vi "update the test result table_bakcup.vi"(6 "Bool引用句柄":refnum<vi>, 7 "Test Result":string[](array[string]), 8 "数组":string[][](array[string]), 9 "Test Start Time":string, 10 "Test Table":refnum<vi>, 11 "LED":T1) -> ()   [LabVIEW 2016]
uses:
  <vilib>/Utility/miscctls.llb/LVRowAndColumnTypeDef.ctl
  Global Variables/Pacemaker ASIC Test_Save_SN Globals.vi
  Global Variables/Pacemaker ASIC Test_Config Globals.vi
  <vilib>/Utility/file.llb/Write Delimited Spreadsheet (string).vi
panel:
  in  "Test Unit Information":string[][](array[string])=[["Module", "SRN"], ["Software", "V01"]]
  in  "清除原有数据":bool
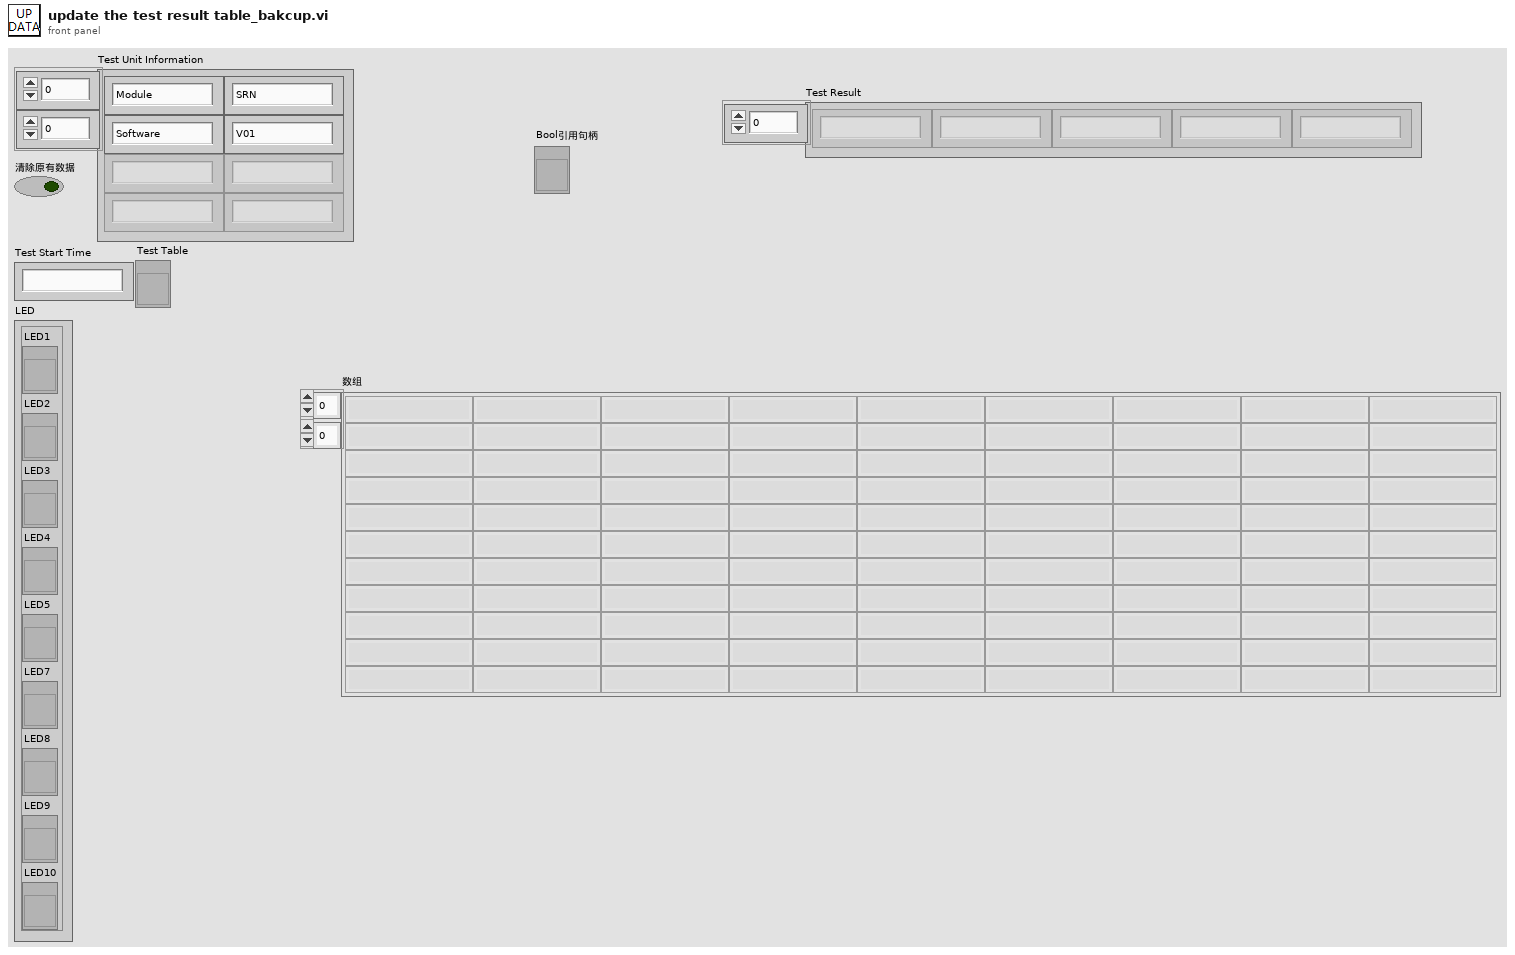
[diagram p1: front panel]
types:
  T1 = cluster{"LED1":refnum<vi>, "LED2":refnum<vi>, "LED3":refnum<vi>, "LED4":refnum<vi>, "LED5":refnum<vi>, "LED7":refnum<vi>, "LED8":refnum<vi>, "LED9":refnum<vi>, "LED10":refnum<vi>}
  T2 = typedef "LVRowAndColumnTypeDef.ctl" = cluster{"Row":i32, "Column":i32}
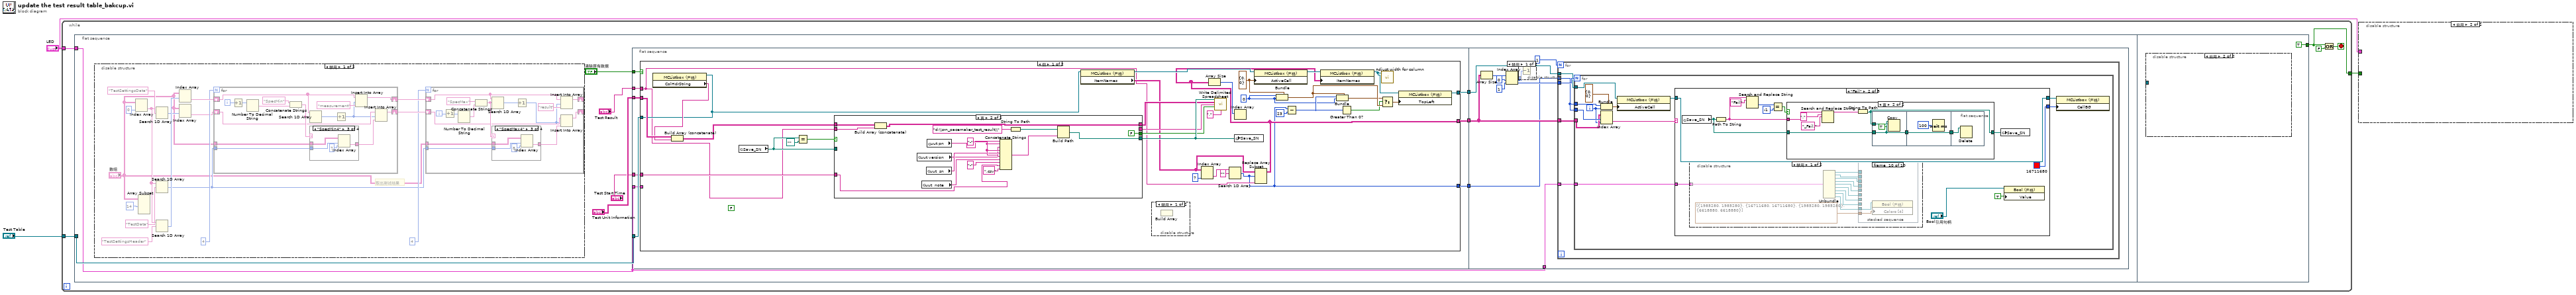
[diagram p0: block diagram]
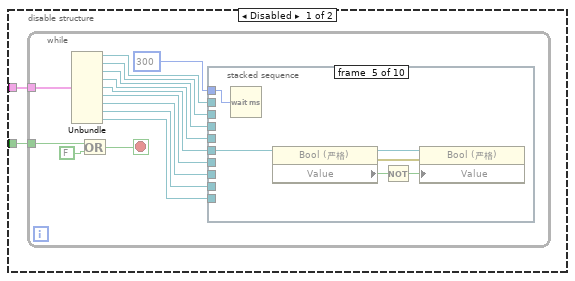
[diagram p2: hidden frame]
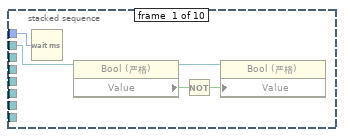
[diagram p3: hidden frame]
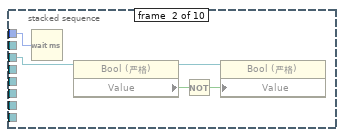
[diagram p4: hidden frame]
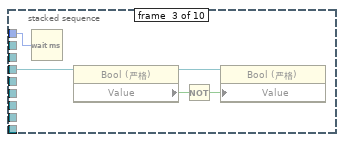
[diagram p5: hidden frame]
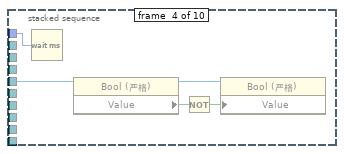
[diagram p6: hidden frame]
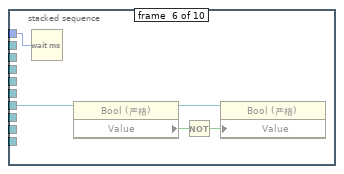
[diagram p7: hidden frame]
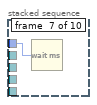
[diagram p8: hidden frame]
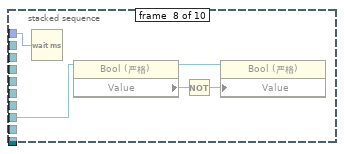
[diagram p9: hidden frame]
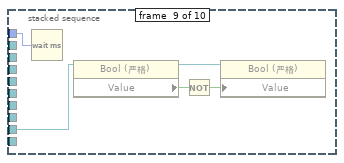
[diagram p10: hidden frame]
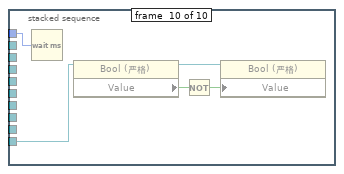
[diagram p11: hidden frame]
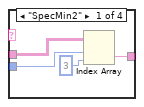
[diagram p12: hidden frame]
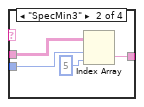
[diagram p13: hidden frame]
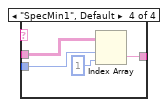
[diagram p14: hidden frame]
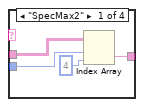
[diagram p15: hidden frame]
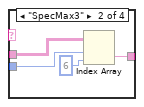
[diagram p16: hidden frame]
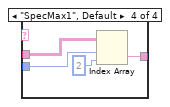
[diagram p17: hidden frame]
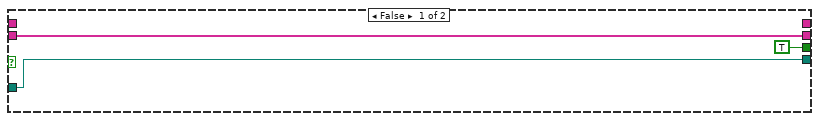
[diagram p20: hidden frame]
diagram:
  n1 = while {
    tunnel: "Test Table" -> [w8]
    tunnel: [w5] -> w3
    tunnel: "LED" -> [w4]
    stop <- w6 stop-if-true
    n2 = flat-sequence {
      tunnel: w8 -> [w14]
      tunnel: w4 -> [w13]
      tunnel: [TRUE] -> w5
      frame #0 {
        n3 = disable-structure shown="禁用" {
          frame Disabled {
            # "取出测试结果"
            n4 = Index Array(array="数组", index (col)=0 ("禁用的索引 (列)")) -> (element=w22:string[])  [unwired: 1 in]
            n5 = Array Subset(array="数组", length (row)=14 ("长度")) -> ()  [unwired: 3 in, 1 out]
            n6 = Search 1D Array(1D array=w22, element="TestSettingsData" ("元素")) -> (index of element=w23:i32)  [unwired: 1 in]
            n7 = Search 1D Array(1D array=w22, element="TestData" ("元素")) -> (index of element=w20:i32)  [unwired: 1 in]
            n8 = Search 1D Array(1D array=w22, element="TestSettingsHeader" ("元素")) -> (index of element=w25:i32)  [unwired: 1 in]
            n9 = Index Array(array="数组", index (row)=w25) -> (element=w33:string[])  [unwired: 1 in]
            n10 = Index Array(array="数组", index (row)=w23) -> (element=w31:string[])  [unwired: 1 in]
            n11 = for {
              N: 4 -> [_]
              shift-right: [w42] -> w30
              shift-left: w33 -> [w43]
              shift-right: [w39] -> w29
              shift-left: w31 -> [w40]
              tunnel: "数组" -> [w35]
              tunnel: w20 -> [w34]
              i -> [w47]
              n12 = Increment(x=w47) -> (x+1=w46:i32)
              n13 = Number To Decimal String(number=w46) -> (decimal integer string=w45:string)  [unwired: 1 in]
              n14 = Concatenate Strings("SpecMin" ("元素"), w45) -> (w44:string)
              n15 = Search 1D Array(1D array=w43, element=w44) -> (index of element=w41:i32)  [unwired: 1 in]
              n16 = case shown="\"SpecMin4\"" w44 {
                tunnel: w35 -> [w51 w55 w57 w64]
                tunnel: [w50 w53 w59 w62] -> w37
                tunnel: w34 -> [w49 w54 w58 w61]
                frame "SpecMin2" {
                  n17 = Index Array(array=w51, index (row)=w49, index (col)=3) -> (element=w50:string)
                }
                frame "SpecMin3" {
                  n18 = Index Array(array=w55, index (row)=w54, index (col)=5) -> (element=w53:string)
                }
                frame "SpecMin4" {
                  n19 = Index Array(array=w57, index (row)=w58, index (col)=7) -> (element=w59:string)
                }
                frame "SpecMin1", Default {
                  n20 = Index Array(array=w64, index (row)=w61, index (col)=1) -> (element=w62:string)
                }
              }
              n21 = Increment(x=w41) -> (x+1=w36:i32)
              n22 = Insert Into Array(array=w43, index=w36, new element="measurement" ("新元素/子数组")) -> (w42:string[])
              n23 = Insert Into Array(array=w40, index=w36, new element=w37) -> (w39:string[])
            }
            n24 = for {
              N: 4 -> [_]
              shift-right: [w73] -> _
              shift-left: w30 -> [w74]
              shift-right: [w70] -> _
              shift-left: w29 -> [w71]
              tunnel: "数组" -> [w66]
              tunnel: w20 -> [w65]
              i -> [w78]
              n25 = Increment(x=w78) -> (x+1=w77:i32)
              n26 = Number To Decimal String(number=w77) -> (decimal integer string=w76:string)  [unwired: 1 in]
              n27 = Concatenate Strings("SpecMax" ("元素"), w76) -> (w75:string)
              n28 = Search 1D Array(1D array=w74, element=w75) -> (index of element=w72:i32)  [unwired: 1 in]
              n29 = case shown="\"SpecMax4\"" w75 {
                tunnel: w66 -> [w82 w86 w89 w95]
                tunnel: [w81 w84 w90 w93] -> w68
                tunnel: w65 -> [w80 w85 w88 w92]
                frame "SpecMax2" {
                  n30 = Index Array(array=w82, index (row)=w80, index (col)=4) -> (element=w81:string)
                }
                frame "SpecMax3" {
                  n31 = Index Array(array=w86, index (row)=w85, index (col)=6) -> (element=w84:string)
                }
                frame "SpecMax4" {
                  n32 = Index Array(array=w89, index (row)=w88, index (col)=8) -> (element=w90:string)
                }
                frame "SpecMax1", Default {
                  n33 = Index Array(array=w95, index (row)=w92, index (col)=2) -> (element=w93:string)
                }
              }
              n34 = Increment(x=w72) -> (x+1=w67:i32)
              n35 = Insert Into Array(array=w74, index=w67, new element="result" ("新元素/子数组")) -> (w73:string[])
              n36 = Insert Into Array(array=w71, index=w67, new element=w68) -> (w70:string[])
            }
          }
          frame Enabled {
          }
        }
        n37 = flat-sequence {
          tunnel: "Test Result" -> [w104]
          tunnel: "清除原有数据" -> [w103]
          tunnel: w14 -> [w102]
          tunnel: [w101] -> w17
          tunnel: [w100] -> w16
          tunnel: w13 -> [w99]
          tunnel: "Test Unit Information" -> [w98]
          tunnel: "Test Start Time" -> [w97]
          tunnel: [w96] -> w9
          tunnel: w17 -> [w243]
          tunnel: w16 -> [w242]
          tunnel: w13 -> [w241]
          tunnel: w9 -> [w238]
          frame #0 {
            n38 = case shown="假" w103 {
              tunnel: w104 -> [w107 _]
              tunnel: w102 -> [w112 w179]
              tunnel: [w106 _] -> w101
              tunnel: [w121 w177] -> w100
              tunnel: w99 -> [_ w176]
              tunnel: w98 -> [w134 _]
              tunnel: w97 -> [w113 _]
              tunnel: [w105 _] -> w96
              frame False {
                (unwired) FALSE
                w116 = 0
                w125 = T2 {"Row"=0, "Column"=0} ("活动单元格:活动单元格")
                n39 = property class="MCListbox (严格)"(reference=w112) -> ("ColHdrString"=w114:string[])  [unwired: 1 in, 2 out]
                n40 = Build Array (concatenate)(w134, w114) -> (w135:string[][])
                n41 = global read "Pacemaker ASIC Test_Save_SN Globals.vi" "Save_SN"() -> (w131:path)
                n42 = Equal?(x=w131, y=path "") -> (x = y?=w132:bool)
                n43 = case shown="真" w132 {
                  tunnel: w135 -> [_ w144]
                  tunnel: w131 -> [w140 _]
                  tunnel: [w140 w146] -> w130
                  tunnel: [_ w142] -> w129
                  tunnel: [TRUE FALSE] -> w128
                  tunnel: w107 -> [w138 w143]
                  tunnel: [w138 _] -> w127
                  tunnel: w113 -> [_ w141]
                  frame False {
                  }
                  frame True {
                    w155 = "-"
                    n44 = Build Array (concatenate)(w144, w143) -> (w142:string[][])
                    n45 = global read "Pacemaker ASIC Test_Config Globals.vi" "uut version"() -> (w153:string)
                    n46 = global read "Pacemaker ASIC Test_Config Globals.vi" "uut  note"() -> (w156:string)
                    n47 = global read "Pacemaker ASIC Test_Config Globals.vi" "uut  sn"() -> (w154:string)
                    n48 = global read "Pacemaker ASIC Test_Config Globals.vi" "uut pn"() -> (w152:string)
                    n49 = Concatenate Strings(w152, w155, w153, w155, w154, w155, w156, "-", w141, ".csv" ("字符串")) -> (w148:string)
                    n50 = String To Path(string="d:\\srn_pacemaker_test_result\\" ("字符串")) -> (path=w149:path)
                    n51 = Build Path(base path=w149, name or relative path=w148) -> (appended path=w146:path)
                  }
                }
                n52 = property class="MCListbox (严格)"(reference=w112) -> (reference out=w136:refnum<vi>, "ItemNames"=w108:string[][])  [unwired: 1 in, 1 out]
                n53 = disable-structure shown="禁用" {
                  frame Disabled {
                    n54 = Build Array() -> ()  [unwired: 2 in, 1 out]
                  }
                  frame Enabled {
                  }
                }
                n55 = Index Array(array=w108, index (col)=7 ("禁用的索引 (列)")) -> (element=w110:string[])  [unwired: 1 in]
                n56 = call-poly <vilib>:"Write Delimited Spreadsheet.vi"("file path (dialog if empty)"=w130, "2D data"=w129, "1D data"=w127, "append to file? (new file:F)"=w128, "delimiter (\\t)"="," ("delimiter (\\t)")) -> ()  [unwired: 9 in, 2 out]
                n57 = Search 1D Array(1D array=w110, element="" ("元素")) -> (index of element=w105:i32)  [unwired: 1 in]
                n58 = global write "Pacemaker ASIC Test_Save_SN Globals.vi" "Save_SN"(w130) -> ()
                n59 = property class="MCListbox (严格)"(reference=w136, "ActiveCell"=w125) -> (reference out=w137:refnum<vi>)  [unwired: 1 in, 1 out]
                n60 = Replace Array Subset(array=w108, new element=w107, index (row)=w105) -> (w106:string[][])  [unwired: 1 in]
                n61 = Array Size(array=w106) -> (size(s)=w126:i32[])
                n62 = Index Array(array=w126) -> ()  [unwired: 1 in, 1 out]
                n63 = Bundle(cluster=w125, "Row"=w116, "Column"=w116) -> (w124:T2)
                n64 = Subtract(x=w105, y=23) -> (x-y=w117:i32)
                n65 = property class="MCListbox (严格)"(reference=w137, "ItemNames"=w106) -> (reference out=w120:refnum<vi>)  [unwired: 1 in, 1 out]
                n66 = Bundle(cluster=w124, "Row"=w117, "Column"=w116) -> (w123:T2)
                n67 = Greater Than 0?(x=w117) -> (x > 0?=w118:bool)
                n68 = call "Adjust width for column.vi"("MCListbox引用句柄"=w120) -> ()  [unwired: 11 in]
                n69 = Select(t=w123, s=w118, f=w124) -> (s? t:f=w122:T2)
                n70 = property class="MCListbox (严格)"(reference=w120, "TopLeft"=w122) -> (reference out=w121:refnum<vi>)  [unwired: 1 in, 1 out]
              }
              frame True {
                # "初始化MCListbox到空"
                n71 = property class="MCListbox (严格)"(reference=w179, "ActiveCell"=T2 {"Row"=0, "Column"=0} ("活动单元格:活动单元格")) -> (reference out=w164:refnum<vi>)  [unwired: 1 in, 1 out]
                n72 = property class="MCListbox (严格)"(reference=w164) -> (reference out=w163:refnum<vi>, "ItemNames"=w162:string[][])  [unwired: 1 in, 1 out]
                n73 = Array Size(array=w162) -> (size(s)=w161:i32[])
                n74 = property class="MCListbox (严格)"(reference=w163, "ItemNames"=string[][] [] ("项名")) -> (reference out=w178:refnum<vi>)  [unwired: 1 in, 1 out]
                n75 = Index Array(array=w161, index #1=0 ("索引"), index #2=1 ("索引")) -> (element #1=w159:i32, element #2=w157:i32)
                n76 = for {
                  N: w159 -> [_]
                  tunnel: w178 -> [w224]
                  tunnel: [w223] -> w177
                  tunnel: w157 -> [w222]
                  i -> [w225]
                  n77 = for {
                    N: w222 -> [_]
                    tunnel: w225 -> [w232]
                    tunnel: w224 -> [w229]
                    tunnel: [w228] -> w223
                    i -> [w231]
                    n78 = Bundle(cluster=cluster{i32, i32} {0, 0} ("簇"), w232, w231) -> (w233:cluster{i32, i32})
                    n79 = property class="MCListbox (严格)"(reference=w229, "ActiveCell"=w233) -> (reference out=w226:refnum<vi>)  [unwired: 1 in, 1 out]
                    n80 = disable-structure shown="启用" {
                      disable-tunnel: w226 -> [w236 _]
                      disable-tunnel: [w235 _] -> _
                      disable-tunnel: [w234 _] -> _
                      frame Disabled {
                        n81 = property class="MCListbox (严格)"(reference=w236) -> (reference out=w235:refnum<vi>, "CellBG"=w237:u32)  [unwired: 1 in, 1 out]
                        n82 = Not Equal?(x=w237) -> (x != y?=w234:bool)  [unwired: 1 in]
                      }
                      frame Enabled {
                      }
                    }
                    n83 = property class="MCListbox (严格)"(reference=w226, "CellBG"=u32 16448250) -> (reference out=w228:refnum<vi>)  [unwired: 1 in, 1 out]
                  }
                }
                n84 = Unbundle(w176) -> ("LED1"=w175:refnum<vi>, "LED2"=w174:refnum<vi>, "LED3"=w173:refnum<vi>, "LED4"=w172:refnum<vi>, "LED5"=w171:refnum<vi>, "LED7"=w170:refnum<vi>, "LED8"=w167:refnum<vi>, "LED9"=w168:refnum<vi>, "LED10"=w169:refnum<vi>)
                n85 = stacked-sequence {
                  tunnel: w175 -> [w185 _ _ _ _ _ _ _ _ _]
                  tunnel: w174 -> [_ w189 _ _ _ _ _ _ _ _]
                  tunnel: w173 -> [_ _ w193 _ _ _ _ _ _ _]
                  tunnel: w172 -> [_ _ _ w197 _ _ _ _ _ _]
                  tunnel: w171 -> [_ _ _ _ w201 _ _ _ _ _]
                  tunnel: w170 -> [_ _ _ _ _ w205 _ _ _ _]
                  tunnel: w169 -> [_ _ _ _ _ _ _ _ _ w221]
                  tunnel: w168 -> [_ _ _ _ _ _ _ _ w216 _]
                  tunnel: w167 -> [_ _ _ _ _ _ w209 w213 _ _]
                  tunnel: cluster{u32, u32}[] [{1985280, 1985280}, {65358, 65358}, {1985280, 1985280}, {6618880, 6618880}] ("颜色[4]") -> [w184 w188 w192 w196 w200 w204 w208 w212 w217 w220]
                  tunnel: TRUE -> [w183 w187 w191 w194 w198 w202 w206 w210 w214 w218]
                  frame #0 {
                    n86 = property class="Bool (严格)"(reference=w185, "Colors [4]"=w184) -> (reference out=w182:refnum<vi>)  [unwired: 1 in, 1 out]
                    n87 = property class="Bool (严格)"(reference=w182, "Value"=w183) -> ()  [unwired: 1 in, 2 out]
                  }
                  frame #1 {
                    n88 = property class="Bool (严格)"(reference=w189, "Colors [4]"=w188) -> (reference out=w186:refnum<vi>)  [unwired: 1 in, 1 out]
                    n89 = property class="Bool (严格)"(reference=w186, "Value"=w187) -> ()  [unwired: 1 in, 2 out]
                  }
                  frame #2 {
                    n90 = property class="Bool (严格)"(reference=w193, "Colors [4]"=w192) -> (reference out=w190:refnum<vi>)  [unwired: 1 in, 1 out]
                    n91 = property class="Bool (严格)"(reference=w190, "Value"=w191) -> ()  [unwired: 1 in, 2 out]
                  }
                  frame #3 {
                    n92 = property class="Bool (严格)"(reference=w197, "Colors [4]"=w196) -> (reference out=w195:refnum<vi>)  [unwired: 1 in, 1 out]
                    n93 = property class="Bool (严格)"(reference=w195, "Value"=w194) -> ()  [unwired: 1 in, 2 out]
                  }
                  frame #4 {
                    n94 = property class="Bool (严格)"(reference=w201, "Colors [4]"=w200) -> (reference out=w199:refnum<vi>)  [unwired: 1 in, 1 out]
                    n95 = property class="Bool (严格)"(reference=w199, "Value"=w198) -> ()  [unwired: 1 in, 2 out]
                  }
                  frame #5 {
                    n96 = property class="Bool (严格)"(reference=w205, "Colors [4]"=w204) -> (reference out=w203:refnum<vi>)  [unwired: 1 in, 1 out]
                    n97 = property class="Bool (严格)"(reference=w203, "Value"=w202) -> ()  [unwired: 1 in, 2 out]
                  }
                  frame #6 {
                    n98 = property class="Bool (严格)"(reference=w209, "Colors [4]"=w208) -> (reference out=w207:refnum<vi>)  [unwired: 1 in, 1 out]
                    n99 = property class="Bool (严格)"(reference=w207, "Value"=w206) -> ()  [unwired: 1 in, 2 out]
                  }
                  frame #7 {
                    n100 = property class="Bool (严格)"(reference=w213, "Colors [4]"=w212) -> (reference out=w211:refnum<vi>)  [unwired: 1 in, 1 out]
                    n101 = property class="Bool (严格)"(reference=w211, "Value"=w210) -> ()  [unwired: 1 in, 2 out]
                  }
                  frame #8 {
                    n102 = property class="Bool (严格)"(reference=w216, "Colors [4]"=w217) -> (reference out=w215:refnum<vi>)  [unwired: 1 in, 1 out]
                    n103 = property class="Bool (严格)"(reference=w215, "Value"=w214) -> ()  [unwired: 1 in, 2 out]
                  }
                  frame #9 {
                    n104 = property class="Bool (严格)"(reference=w221, "Colors [4]"=w220) -> (reference out=w219:refnum<vi>)  [unwired: 1 in, 1 out]
                    n105 = property class="Bool (严格)"(reference=w219, "Value"=w218) -> ()  [unwired: 1 in, 2 out]
                  }
                }
              }
            }
          }
          frame #1 {
            n106 = Array Size(array=w243) -> (size(s)=w247:i32[])
            n107 = Index Array(array=w247, index #1=0 ("索引"), index #2=1 ("索引")) -> (element #1=w240:i32, element #2=w244:i32)
            n108 = disable-structure shown="禁用" {
              disable-tunnel: w240 -> [w248 _]
              frame Disabled {
                n109 = Decrement(x=w248) -> ()  [unwired: 1 out]
              }
              frame Enabled {
              }
            }
            n110 = for {
              N: 1 -> [_]
              tunnel: w244 -> [w253]
              tunnel: w243 -> [w252]
              tunnel: w242 -> [w251]
              tunnel: w241 -> [w250]
              tunnel: w238 -> [w249]
              n111 = for {
                N: w253 -> [_]
                tunnel: w249 -> [w265]
                tunnel: w252 -> [w264]
                tunnel: w249 -> [w261]
                tunnel: w251 -> [w255]
                tunnel: w250 -> [w254]
                i -> [w260]
                n112 = Bundle(cluster=cluster{i32, i32} {0, 0} ("簇"), w261, w260) -> (w262:cluster{i32, i32})
                n113 = Index Array(array=w264, index (row)=w265, index (col)=w260) -> (element=w263:string)
                n114 = property class="MCListbox (严格)"(reference=w255, "ActiveCell"=w262) -> (reference out=w259:refnum<vi>)  [unwired: 1 in, 1 out]
                n115 = case shown="\"Fail\"" w263 {
                  tunnel: w259 -> [w267 w279 w327]
                  tunnel: [w267 w279 w327] -> w258
                  tunnel: [u32 6618880 u32 16711680 u32 16448250] -> w256
                  tunnel: w254 -> [_ w277 _]
                  frame "Pass" {
                  }
                  frame "Fail" {
                    n116 = global read "Pacemaker ASIC Test_Save_SN Globals.vi" "Save_SN"() -> (w270:path)
                    n117 = disable-structure shown="禁用" {
                      disable-tunnel: w277 -> [w281 _]
                      frame Disabled {
                        n118 = Unbundle(w281) -> ("LED1"=w290:refnum<vi>, "LED2"=w289:refnum<vi>, "LED3"=w288:refnum<vi>, "LED4"=w287:refnum<vi>, "LED5"=w286:refnum<vi>, "LED7"=w285:refnum<vi>, "LED8"=w282:refnum<vi>, "LED9"=w283:refnum<vi>, "LED10"=w284:refnum<vi>)
                        n119 = stacked-sequence {
                          tunnel: w290 -> [w292 _ _ _ _ _ _ _ _ _]
                          tunnel: w289 -> [_ w294 _ _ _ _ _ _ _ _]
                          tunnel: w288 -> [_ _ w296 _ _ _ _ _ _ _]
                          tunnel: w287 -> [_ _ _ w298 _ _ _ _ _ _]
                          tunnel: w286 -> [_ _ _ _ w300 _ _ _ _ _]
                          tunnel: w285 -> [_ _ _ _ _ w302 _ _ _ _]
                          tunnel: w284 -> [_ _ _ _ _ _ _ _ _ w310]
                          tunnel: w283 -> [_ _ _ _ _ _ _ _ w307 _]
                          tunnel: w282 -> [_ _ _ _ _ _ w304 w306 _ _]
                          tunnel: cluster{u32, u32}[] [{1985280, 1985280}, {16711680, 16711680}, {1985280, 1985280}, {6618880, 6618880}] ("颜色[4]") -> [w291 w293 w295 w297 w299 w301 w303 w305 w308 w309]
                          frame #0 {
                            n120 = property class="Bool (严格)"(reference=w292, "Colors [4]"=w291) -> ()  [unwired: 1 in, 2 out]
                          }
                          frame #1 {
                            n121 = property class="Bool (严格)"(reference=w294, "Colors [4]"=w293) -> ()  [unwired: 1 in, 2 out]
                          }
                          frame #2 {
                            n122 = property class="Bool (严格)"(reference=w296, "Colors [4]"=w295) -> ()  [unwired: 1 in, 2 out]
                          }
                          frame #3 {
                            n123 = property class="Bool (严格)"(reference=w298, "Colors [4]"=w297) -> ()  [unwired: 1 in, 2 out]
                          }
                          frame #4 {
                            n124 = property class="Bool (严格)"(reference=w300, "Colors [4]"=w299) -> ()  [unwired: 1 in, 2 out]
                          }
                          frame #5 {
                            n125 = property class="Bool (严格)"(reference=w302, "Colors [4]"=w301) -> ()  [unwired: 1 in, 2 out]
                          }
                          frame #6 {
                            n126 = property class="Bool (严格)"(reference=w304, "Colors [4]"=w303) -> ()  [unwired: 1 in, 2 out]
                          }
                          frame #7 {
                            n127 = property class="Bool (严格)"(reference=w306, "Colors [4]"=w305) -> ()  [unwired: 1 in, 2 out]
                          }
                          frame #8 {
                            n128 = property class="Bool (严格)"(reference=w307, "Colors [4]"=w308) -> ()  [unwired: 1 in, 2 out]
                          }
                          frame #9 {
                            n129 = property class="Bool (严格)"(reference=w310, "Colors [4]"=w309) -> ()  [unwired: 1 in, 2 out]
                          }
                        }
                      }
                      frame Enabled {
                      }
                    }
                    n130 = Path To String(path=w270) -> (string=w272:string)
                    n131 = Search and Replace String(input string=w272, search string="Fail" ("搜索字符串")) -> (offset past replacement=w275:i32)  [unwired: 6 in, 3 out]
                    n132 = Equal?(x=w275, y=-1) -> (x = y?=w273:bool)
                    n133 = case shown="真" w273 {
                      tunnel: w272 -> [_ w315]
                      tunnel: [w311 w318] -> w271
                      tunnel: w270 -> [w311 w319]
                      frame False {
                      }
                      frame True {
                        n134 = Search and Replace String(input string=w315, search string="." ("搜索字符串"), replace string="_Fail." ("字符串")) -> (result string=w312:string)  [unwired: 5 in, 3 out]
                        n135 = String To Path(string=w312) -> (path=w318:path)
                        n136 = flat-sequence {
                          tunnel: w319 -> [w321]
                          tunnel: w318 -> [w322]
                          tunnel: [w321] -> w316
                          tunnel: [w323] -> w317
                          tunnel: w316 -> [w323]
                          tunnel: w317 -> [w325]
                          frame #0 {
                            n137 = Copy(9:TRUE ("覆盖(F)"), 10:w322, 11:w321) -> ()  [unwired: 2 in, 3 out]
                          }
                          frame #1 {
                            n138 = Wait (ms)(milliseconds to wait=u32 100 ("等待时间（毫秒）")) -> ()  [unwired: 1 out]
                          }
                          frame #2 {
                            n139 = Delete(path (use dialog)=w325) -> ()  [unwired: 4 in, 3 out]
                          }
                        }
                      }
                    }
                    n140 = global write "Pacemaker ASIC Test_Save_SN Globals.vi" "Save_SN"(w271) -> ()
                    n141 = property class="Bool (严格)"(reference="Bool引用句柄", "Value"=TRUE ("值")) -> ()  [unwired: 1 in, 2 out]
                  }
                  frame Default {
                  }
                }
                n142 = property class="MCListbox (严格)"(reference=w258, "CellBG"=w256) -> ()  [unwired: 1 in, 2 out]
              }
            }
          }
        }
      }
      frame #1 {
        n143 = disable-structure shown="启用" {
          disable-tunnel: _ -> [w329 _]
          frame Disabled {
            n144 = stacked-sequence {
              tunnel: w329 -> [w335 w341]
              tunnel: 100 -> [w332 w338]
              tunnel: [_ w337] -> w330
              frame #0 {
                w334 = TRUE
                n145 = Wait (ms)(milliseconds to wait=w332) -> ()  [unwired: 1 out]
                n146 = Variant To Data(type=w334, Variant=w334) -> (data=w333:bool)  [unwired: 1 in, 1 out]
                n147 = invoke class="VI (严格)" method="Ctrl Val.Set"(reference=w335, "Control Name"="Blinking" ("控件名"), "Value"=w333) -> ()  [unwired: 2 in, 5 out]
              }
              frame #1 {
                w340 = FALSE
                n148 = Wait (ms)(milliseconds to wait=w338) -> ()  [unwired: 1 out]
                n149 = Variant To Data(type=w340, Variant=w340) -> (data=w339:bool)  [unwired: 1 in, 1 out]
                n150 = invoke class="VI (严格)" method="Ctrl Val.Set"(reference=w341, "Control Name"="Blinking" ("控件名"), "Value"=w339) -> (reference out=w337:refnum<vi>)  [unwired: 2 in, 4 out]
              }
            }
            n151 = Close Reference(reference=w330) -> ()  [unwired: 1 in, 1 out]
          }
          frame Enabled {
          }
        }
      }
    }
    n152 = Or(x=w5, y=FALSE) -> (x .or. y?=w6:bool)
  }
  n153 = disable-structure shown="启用" {
    disable-tunnel: w3 -> [w344 _]
    disable-tunnel: "LED" -> [w343 _]
    frame Disabled {
      n154 = while {
        tunnel: w343 -> [w358]
        tunnel: w344 -> [w347]
        stop <- w346 stop-if-true
        n155 = Unbundle(w358) -> ("LED1"=w357:refnum<vi>, "LED2"=w355:refnum<vi>, "LED3"=w354:refnum<vi>, "LED4"=w353:refnum<vi>, "LED5"=w352:refnum<vi>, "LED7"=w351:refnum<vi>, "LED8"=w348:refnum<vi>, "LED9"=w349:refnum<vi>, "LED10"=w350:refnum<vi>)
        n156 = Or(x=w347, y=FALSE) -> (x .or. y?=w346:bool)
        n157 = stacked-sequence {
          tunnel: w357 -> [w363 _ _ _ _ _ _ _ _ _]
          tunnel: 300 -> [w359 w366 w369 w374 w380 w387 w390 w393 w396 w403]
          tunnel: w355 -> [_ w368 _ _ _ _ _ _ _ _]
          tunnel: w354 -> [_ _ w370 _ _ _ _ _ _ _]
          tunnel: w353 -> [_ _ _ w378 _ _ _ _ _ _]
          tunnel: w352 -> [_ _ _ _ w379 _ _ _ _ _]
          tunnel: w351 -> [_ _ _ _ _ w386 _ _ _ _]
          tunnel: w350 -> [_ _ _ _ _ _ _ _ _ w405]
          tunnel: w349 -> [_ _ _ _ _ _ _ _ w400 _]
          tunnel: w348 -> [_ _ _ _ _ _ _ w395 _ _]
          frame #0 {
            n158 = Wait (ms)(milliseconds to wait=w359) -> ()  [unwired: 1 out]
            n159 = property class="Bool (严格)"(reference=w363) -> (reference out=w362:refnum<vi>, "Value"=w361:bool)  [unwired: 1 in, 1 out]
            n160 = Not(x=w361) -> (.not. x?=w360:bool)
            n161 = property class="Bool (严格)"(reference=w362, "Value"=w360) -> ()  [unwired: 1 in, 2 out]
          }
          frame #1 {
            n162 = Wait (ms)(milliseconds to wait=w366) -> ()  [unwired: 1 out]
            n163 = property class="Bool (严格)"(reference=w368) -> (reference out=w367:refnum<vi>, "Value"=w365:bool)  [unwired: 1 in, 1 out]
            n164 = Not(x=w365) -> (.not. x?=w364:bool)
            n165 = property class="Bool (严格)"(reference=w367, "Value"=w364) -> ()  [unwired: 1 in, 2 out]
          }
          frame #2 {
            n166 = Wait (ms)(milliseconds to wait=w369) -> ()  [unwired: 1 out]
            n167 = property class="Bool (严格)"(reference=w370) -> (reference out=w371:refnum<vi>, "Value"=w373:bool)  [unwired: 1 in, 1 out]
            n168 = Not(x=w373) -> (.not. x?=w372:bool)
            n169 = property class="Bool (严格)"(reference=w371, "Value"=w372) -> ()  [unwired: 1 in, 2 out]
          }
          frame #3 {
            n170 = Wait (ms)(milliseconds to wait=w374) -> ()  [unwired: 1 out]
            n171 = property class="Bool (严格)"(reference=w378) -> (reference out=w377:refnum<vi>, "Value"=w376:bool)  [unwired: 1 in, 1 out]
            n172 = Not(x=w376) -> (.not. x?=w375:bool)
            n173 = property class="Bool (严格)"(reference=w377, "Value"=w375) -> ()  [unwired: 1 in, 2 out]
          }
          frame #4 {
            n174 = Wait (ms)(milliseconds to wait=w380) -> ()  [unwired: 1 out]
            n175 = property class="Bool (严格)"(reference=w379) -> (reference out=w384:refnum<vi>, error out=w383:errorcluster, "Value"=w382:bool)  [unwired: 1 in]
            n176 = Not(x=w382) -> (.not. x?=w381:bool)
            n177 = property class="Bool (严格)"(reference=w384, error in=w383, "Value"=w381) -> ()  [unwired: 2 out]
          }
          frame #5 {
            n178 = Wait (ms)(milliseconds to wait=w387) -> ()  [unwired: 1 out]
            n179 = property class="Bool (严格)"(reference=w386) -> (reference out=w385:refnum<vi>, "Value"=w389:bool)  [unwired: 1 in, 1 out]
            n180 = Not(x=w389) -> (.not. x?=w388:bool)
            n181 = property class="Bool (严格)"(reference=w385, "Value"=w388) -> ()  [unwired: 1 in, 2 out]
          }
          frame #6 {
            n182 = Wait (ms)(milliseconds to wait=w390) -> ()  [unwired: 1 out]
          }
          frame #7 {
            n183 = Wait (ms)(milliseconds to wait=w393) -> ()  [unwired: 1 out]
            n184 = property class="Bool (严格)"(reference=w395) -> (reference out=w394:refnum<vi>, "Value"=w392:bool)  [unwired: 1 in, 1 out]
            n185 = Not(x=w392) -> (.not. x?=w391:bool)
            n186 = property class="Bool (严格)"(reference=w394, "Value"=w391) -> ()  [unwired: 1 in, 2 out]
          }
          frame #8 {
            n187 = Wait (ms)(milliseconds to wait=w396) -> ()  [unwired: 1 out]
            n188 = property class="Bool (严格)"(reference=w400) -> (reference out=w399:refnum<vi>, "Value"=w398:bool)  [unwired: 1 in, 1 out]
            n189 = Not(x=w398) -> (.not. x?=w397:bool)
            n190 = property class="Bool (严格)"(reference=w399, "Value"=w397) -> ()  [unwired: 1 in, 2 out]
          }
          frame #9 {
            n191 = Wait (ms)(milliseconds to wait=w403) -> ()  [unwired: 1 out]
            n192 = property class="Bool (严格)"(reference=w405) -> (reference out=w404:refnum<vi>, "Value"=w402:bool)  [unwired: 1 in, 1 out]
            n193 = Not(x=w402) -> (.not. x?=w401:bool)
            n194 = property class="Bool (严格)"(reference=w404, "Value"=w401) -> ()  [unwired: 1 in, 2 out]
          }
        }
      }
    }
    frame Enabled {
    }
  }
